vi "BSTMultipleNumericLimitTest.vi"() -> (0 "error out":errorcluster, 1 "Report Text":string, 2 "Measurements":dbl[](array[numeric])=[24.0, -1.0] format="%.2f")   [LabVIEW 2013]
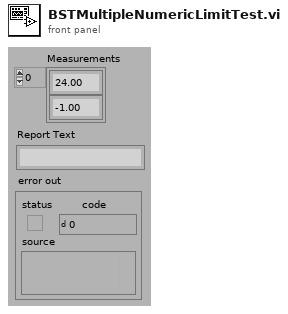
[diagram p1: front panel]
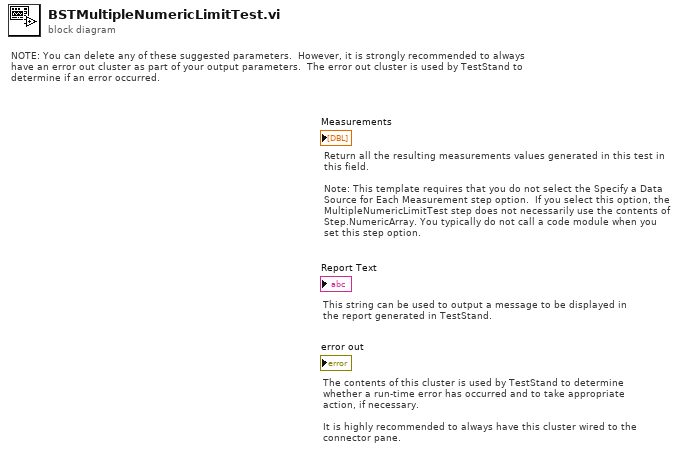
[diagram p0: block diagram]
diagram:
  # "The contents of this cluster is used by TestStand to determine whether a run-time error has occurred and to take appropriate action, if necessary.\n\nIt is highly recommended to always have this cluster wired to the connector pane."
  # "This string can be used to output a message to be displayed in the report generated in TestStand."
  # "NOTE: You can delete any of these suggested parameters.  However, it is strongly recommended to always have an error out cluster as part of your output parameters.  The error out cluster is used by TestStand to determine if an error occurred."
  # "Return all the resulting measurements values generated in this test in this field.\n\nNote: This template requires that you do not select the Specify a Data Source for Each Measurement step option.  If you select this option, the MultipleNumericLimitTest step does not necessarily use the contents of Step.NumericArray. You typically do not call a code module when you set this step option."
